vi "save data link.vi"() -> ()   [LabVIEW 2013]
panel:
  in  "udl name":path=path "db.udl"
  in  "mdb name":path=path "db.mdb"
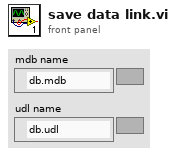
[diagram p1: front panel]
types:
  T1 = enum16{"open", "replace", "create", "open or create", "replace or create", "replace or create with confirmation"}
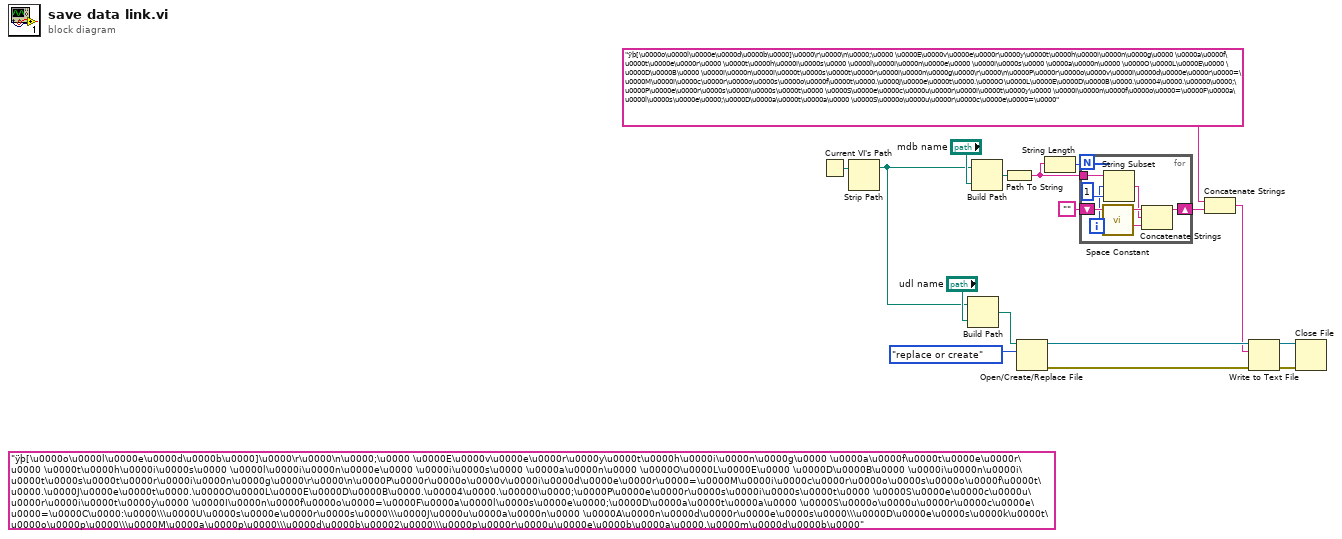
[diagram p0: block diagram]
diagram:
  (unwired) "ÿþ[\u0000o\u0000l\u0000e\u0000d\u0000b\u0000]\u0000\r\u0000\n\u0000;\u0000 \u0000E\u0000v\u0000e\u0000r\u0000y\u0000t\u0000h\u0000i\u0000n\u0000g\u0000 \u0000a\u0000f\u0000t\u0000e\u0000r\u0000 \u0000t\u0000h\u0000i\u0000s\u0000 \u0000l\u0000i\u0000n\u0000e\u0000 \u0000i\u0000s\u0000 \u0000a\u0000n\u0000 \u0000O\u0000L\u0000E\u0000 \u0000D\u0000B\u0000 \u0000i\u0000n\u0000i\u0000t\u0000s\u0000t\u0000r\u0000i\u0000n\u0000g\u0000\r\u0000\n\u0000P\u0000r\u0000o\u0000v\u0000i\u0000d\u0000e\u0000r\u0000=\u0000M\u0000i\u0000c\u0000r\u0000o\u0000s\u0000o\u0000f\u0000t\u0000.\u0000J\u0000e\u0000t\u0000.\u0000O\u0000L\u0000E\u0000D\u0000B\u0000.\u00004\u0000.\u00000\u0000;\u0000P\u0000e\u0000r\u0000s\u0000i\u0000s\u0000t\u0000 \u0000S\u0000e\u0000c\u0000u\u0000r\u0000i\u0000t\u0000y\u0000 \u0000I\u0000n\u0000f\u0000o\u0000=\u0000F\u0000a\u0000l\u0000s\u0000e\u0000;\u0000D\u0000a\u0000t\u0000a\u0000 \u0000S\u0000o\u0000u\u0000r\u0000c\u0000e\u0000=\u0000C\u0000:\u0000\\\u0000U\u0000s\u0000e\u0000r\u0000s\u0000\\\u0000J\u0000u\u0000a\u0000n\u0000 \u0000A\u0000n\u0000d\u0000r\u0000e\u0000s\u0000\\\u0000D\u0000e\u0000s\u0000k\u0000t\u0000o\u0000p\u0000\\\u0000M\u0000a\u0000p\u0000\\\u0000d\u0000b\u00002\u0000\\\u0000p\u0000r\u0000u\u0000e\u0000b\u0000a\u0000.\u0000m\u0000d\u0000b\u0000" ("text")
  n1 = Current VI's Path() -> (path=w14:path)
  n2 = Strip Path(path=w14) -> (stripped path=w4:path)  [unwired: 1 out]
  n3 = Build Path(base path=w4, name or relative path="udl name") -> (appended path=w5:path)
  n4 = Build Path(base path=w4, name or relative path="mdb name") -> (appended path=w10:path)
  n5 = Path To String(path=w10) -> (string=w8:string)
  n6 = Open/Create/Replace File(file path (use dialog)=w5, operation (0:open)=T1."replace or create") -> (refnum out=w11:refnum<file>, error out=w12:errorcluster)  [unwired: 4 in, 1 out]
  n7 = String Length(string=w8) -> (length=w9:i32)
  n8 = for {
    N: w9 -> [_]
    tunnel: w8 -> [w24]
    shift-right: [w21] -> w3
    shift-left: "" -> [w22]
    i -> [w18]
    n9 = call <vilib>:"Space Constant.vi"() -> ("String"=w23:string)
    n10 = String Subset(string=w24, offset (0)=w18, length (rest)=1 ("length (rest)")) -> (substring=w19:string)
    n11 = Concatenate Strings(w22, w19, w23) -> (w21:string)
  }
  n12 = Concatenate Strings("ÿþ[\u0000o\u0000l\u0000e\u0000d\u0000b\u0000]\u0000\r\u0000\n\u0000;\u0000 \u0000E\u0000v\u0000e\u0000r\u0000y\u0000t\u0000h\u0000i\u0000n\u0000g\u0000 \u0000a\u0000f\u0000t\u0000e\u0000r\u0000 \u0000t\u0000h\u0000i\u0000s\u0000 \u0000l\u0000i\u0000n\u0000e\u0000 \u0000i\u0000s\u0000 \u0000a\u0000n\u0000 \u0000O\u0000L\u0000E\u0000 \u0000D\u0000B\u0000 \u0000i\u0000n\u0000i\u0000t\u0000s\u0000t\u0000r\u0000i\u0000n\u0000g\u0000\r\u0000\n\u0000P\u0000r\u0000o\u0000v\u0000i\u0000d\u0000e\u0000r\u0000=\u0000M\u0000i\u0000c\u0000r\u0000o\u0000s\u0000o\u0000f\u0000t\u0000.\u0000J\u0000e\u0000t\u0000.\u0000O\u0000L\u0000E\u0000D\u0000B\u0000.\u00004\u0000.\u00000\u0000;\u0000P\u0000e\u0000r\u0000s\u0000i\u0000s\u0000t\u0000 \u0000S\u0000e\u0000c\u0000u\u0000r\u0000i\u0000t\u0000y\u0000 \u0000I\u0000n\u0000f\u0000o\u0000=\u0000F\u0000a\u0000l\u0000s\u0000e\u0000;\u0000D\u0000a\u0000t\u0000a\u0000 \u0000S\u0000o\u0000u\u0000r\u0000c\u0000e\u0000=\u0000" ("text"), w3) -> (w1:string)
  n13 = Write to Text File(file (use dialog)=w11, text=w1, error in=w12) -> (refnum out=w16:refnum<file>, error out=w17:errorcluster)  [unwired: 1 in, 1 out]
  n14 = Close File(refnum=w16, error in=w17) -> ()  [unwired: 2 out]
